vi "Initialize Configuration.vi"(8 "error in (no error)":errorcluster, 10 "framework configuration in":T1, 11 "VeriStand Data Sharing Framework in":refnum<class "VeriStand Data Sharing Framework.lvclass">) -> (0 "error out":errorcluster, 2 "framework configuration out":T1, 3 "VeriStand Data Sharing Framework out":refnum<class "VeriStand Data Sharing Framework.lvclass">)   [LabVIEW 2017, in "Data Sharing Custom Device Engine.lvlib" / "VeriStand Data Sharing Framework.lvclass"]
uses:
  VeriStand Data Sharing Framework.lvclass
  Builds/Data Sharing Framework/Current/Core/DSF Core.lvlibp/DSF Configuration API/Public/Controls/DSF Engine Framework Configuration.ctl
  Builds/Data Sharing Framework/Current/Core/DSF Core.lvlibp/DSF Configuration API/Public/Controls/DSF Engine Plugin Configuration.ctl
  Builds/Data Sharing Framework/Current/Core/DSF Core.lvlibp/DSF Configuration API/Public/Controls/DSF Timing Info.ctl
  Builds/Data Sharing Framework/Current/Core/DSF Core.lvlibp/DSF Configuration API/Public/Controls/DSF Engine Plugin Thread Configuration.ctl
  Builds/Data Sharing Framework/Current/Core/DSF Core.lvlibp/DSF Configuration API/Public/Controls/DSF Settings Info.ctl
  Builds/Data Sharing Framework/Current/Core/DSF Core.lvlibp/DSF Configuration API/Public/Controls/DSF Engine Transfer Group Configuration.ctl
  Builds/Data Sharing Framework/Current/Core/DSF Core.lvlibp/DSF Configuration API/Public/Controls/DSF Direction.ctl
  Builds/Data Sharing Framework/Current/Core/DSF Core.lvlibp/DSF Configuration API/Public/Controls/DSF Engine Transfer Configuration.ctl
  Builds/Data Sharing Framework/Current/Core/DSF Core.lvlibp/DSF Configuration API/Public/Controls/DSF Byte Order.ctl
  Builds/Data Sharing Framework/Current/Core/DSF Core.lvlibp/DSF Configuration API/Public/Controls/DSF Engine Channel Configuration.ctl
  Builds/Data Sharing Framework/Current/Core/DSF Core.lvlibp/DSF Configuration API/Public/Controls/DSF Data Type.ctl
  VeriStand Data Sharing Framework.lvclass/VeriStand Data Sharing Framework.ctl
  <vilib>/NI Veristand/Custom Device API/Data Access Type.ctl
  Builds/Data Sharing Framework/Current/Core/DSF Core.lvlibp/DSF Configuration API/Public/Channel Count (Transfer).vi
  <vilib>/NI Veristand/Custom Device API/Custom Device API.lvlib
  Builds/Data Sharing Framework/Current/Core/DSF Core.lvlibp
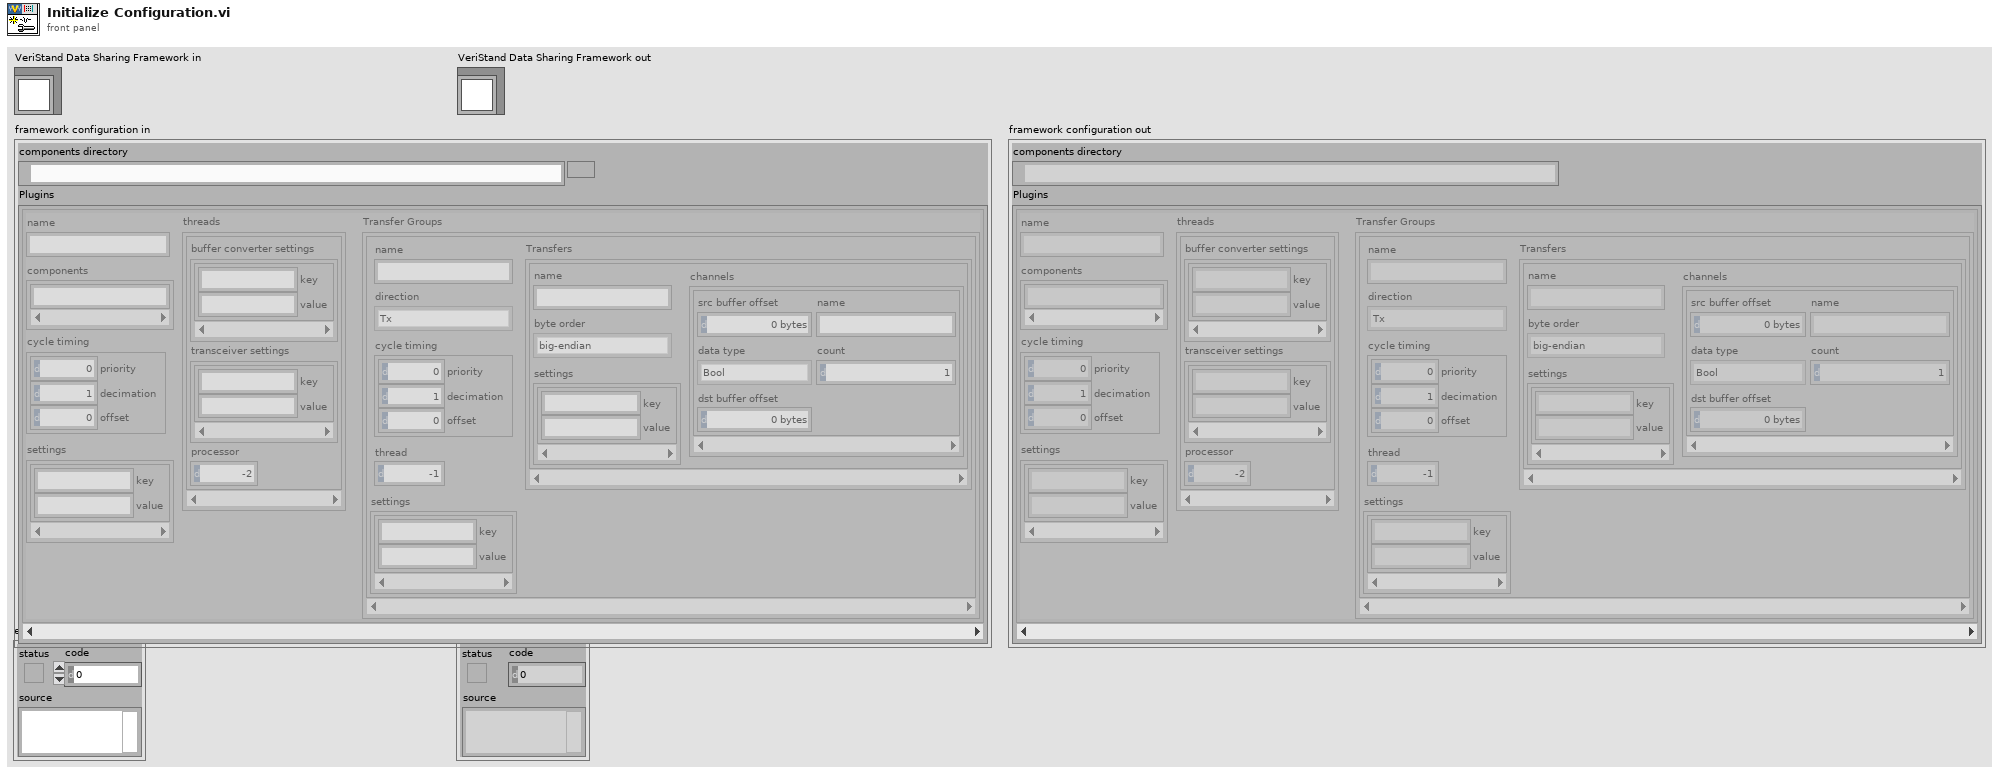
[diagram p1: front panel]
types:
  T1 = typedef "DSF Core.lvlibp/DSF Engine Framework Configuration.ctl" = cluster{"components directory":path, "Plugins":T2[]}
  T2 = typedef "DSF Core.lvlibp/DSF Engine Plugin Configuration.ctl" = cluster{"name":string, "components":string[], "cycle timing":T3, "threads":T4[], "Transfer Groups":T6[], "settings":T5}
  T3 = typedef "DSF Core.lvlibp/DSF Timing Info.ctl" = cluster{"priority":u64, "decimation":u64, "offset":u64}
  T4 = typedef "DSF Core.lvlibp/DSF Engine Plugin Thread Configuration.ctl" = cluster{"buffer converter settings":T5, "transceiver settings":T5, "processor":i32}
  T5 = typedef "DSF Core.lvlibp/DSF Settings Info.ctl" = cluster{"key":string, "value":string}[]
  T6 = typedef "DSF Core.lvlibp/DSF Engine Transfer Group Configuration.ctl" = cluster{"name":string, "direction":T7, "cycle timing":T3, "thread":i32, "settings":T5, "Transfers":T8[]}
  T7 = typedef "DSF Core.lvlibp/DSF Direction.ctl" = enum8{"Tx", "Rx"}
  T8 = typedef "DSF Core.lvlibp/DSF Engine Transfer Configuration.ctl" = cluster{"name":string, "byte order":T9, "channels":T10[], "settings":T5}
  T9 = typedef "DSF Core.lvlibp/DSF Byte Order.ctl" = enum8{"big-endian", "little-endian"}
  T10 = typedef "DSF Core.lvlibp/DSF Engine Channel Configuration.ctl" = cluster{"src buffer offset":u64, "name":string, "data type":T11, "count":u64, "dst buffer offset":u64}
  T11 = typedef "DSF Core.lvlibp/DSF Data Type.ctl" = enum8{"Bool", "SGL", "DBL", "I8", "I16", "I32", "I64", "U8", "U16", "U32", "U64"}
  T12 = typedef "Custom Device API.lvlib/Data Access Type.ctl" = enum16{"Read", "Write"}
  T13 = typedef "Custom Device API.lvlib/Custom Device Item Ref.ctl" = u64
  T14 = typedef "Custom Device API.lvlib/Block Data Reference.ctl" = cluster{"Data Reference":T15, "Offset":u64, "Length":u64}
  T15 = typedef "Custom Device API.lvlib/Data Reference.ctl" = i32
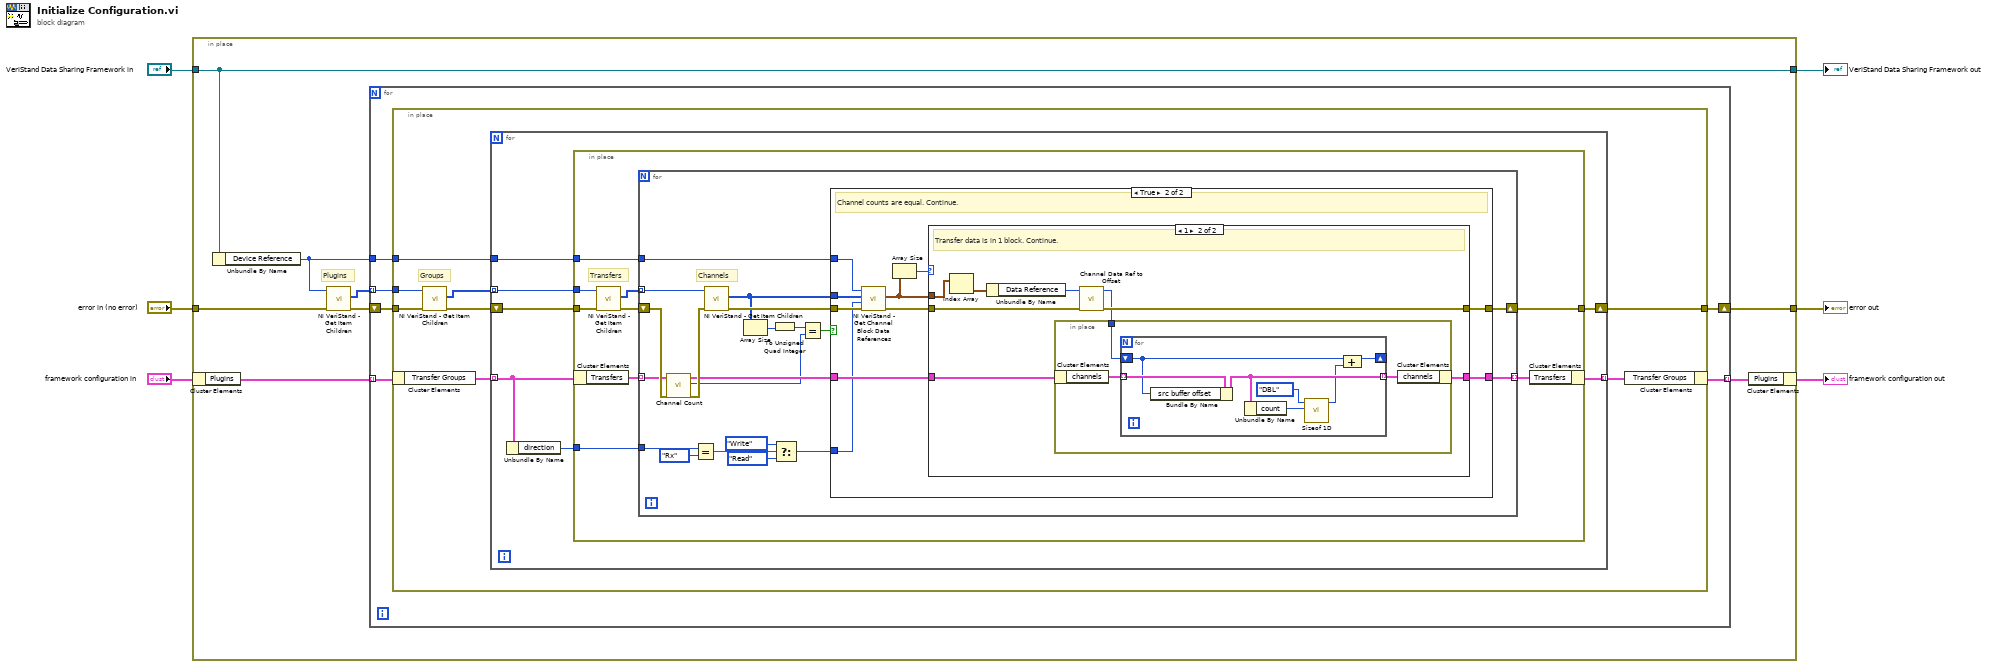
[diagram p0: block diagram]
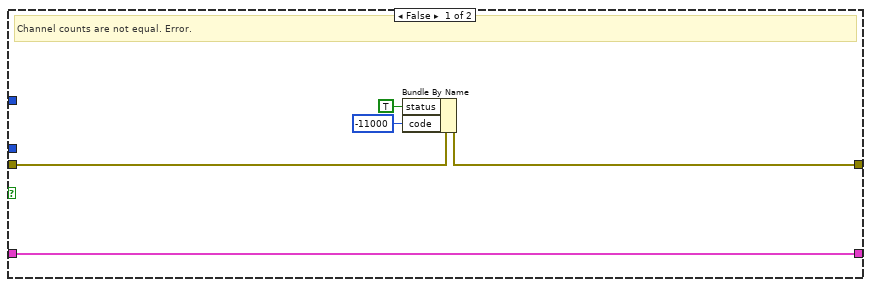
[diagram p2: hidden frame]
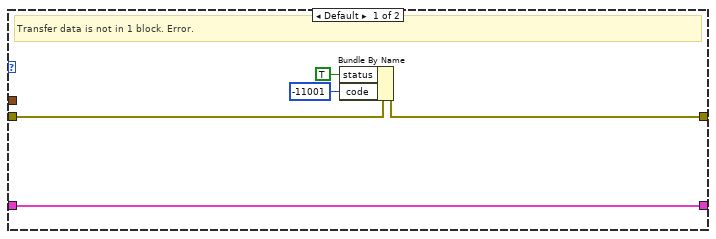
[diagram p3: hidden frame]
diagram:
  n1 = in-place {
    in-place-border: "VeriStand Data Sharing Framework in" -> [w13]
    in-place-border: [w13] -> w5
    in-place-border: "error in (no error)" -> [w8]
    in-place-border: [w7] -> w1
    # "Plugins"
    n2 = in-place-cluster #1("framework configuration in") -> ("Plugins"=w12:T2[])
    n3 = Unbundle By Name(w13) -> ("Device Reference"=w10:T13)
    n4 = call <vilib>:"NI VeriStand - Get Item Children.vi"("error in (no error)"=w8, "Item Ref in"=w10) -> ("error out"=w9:errorcluster, "Child Refs"=w14:T13[])  [unwired: 6 in, 2 out]
    n5 = for {
      tunnel: w14 -> [w18] mode=indexing
      tunnel: w12 -> [w20] mode=indexing
      tunnel: [w19] -> w11 mode=indexing
      tunnel: w10 -> [w17]
      shift-right: [w15] -> w7
      shift-left: w9 -> [w16]
      n6 = in-place {
        in-place-border: w18 -> [w26]
        in-place-border: w17 -> [w24]
        in-place-border: w16 -> [w23]
        in-place-border: [w21] -> w15
        # "Groups"
        n7 = in-place-cluster #2(w20) -> ("Transfer Groups"=w28:T6[])
        n8 = call <vilib>:"NI VeriStand - Get Item Children.vi"("error in (no error)"=w23, "Item Ref in"=w26) -> ("error out"=w22:errorcluster, "Child Refs"=w25:T13[])  [unwired: 6 in, 2 out]
        n9 = for {
          tunnel: w28 -> [w33] mode=indexing
          tunnel: [w35] -> w27 mode=indexing
          tunnel: w25 -> [w34] mode=indexing
          tunnel: w24 -> [w31]
          shift-right: [w29] -> w21
          shift-left: w22 -> [w30]
          n10 = Unbundle By Name(w33) -> ("direction"=w32:T7)
          n11 = in-place {
            in-place-border: w34 -> [w44]
            in-place-border: w32 -> [w41]
            in-place-border: w31 -> [w40]
            in-place-border: w30 -> [w39]
            in-place-border: [w37] -> w29
            # "Transfers"
            n12 = in-place-cluster #3(w33) -> ("Transfers"=w43:T8[])
            n13 = call <vilib>:"NI VeriStand - Get Item Children.vi"("error in (no error)"=w39, "Item Ref in"=w44) -> ("error out"=w38:errorcluster, "Child Refs"=w42:T13[])  [unwired: 6 in, 2 out]
            n14 = for {
              tunnel: w43 -> [w47] mode=indexing
              tunnel: w42 -> [w64] mode=indexing
              tunnel: w41 -> [w62]
              tunnel: w40 -> [w55]
              shift-right: [w46] -> w37
              shift-left: w38 -> [w51]
              tunnel: [w45] -> w36 mode=indexing
              # "Channels"
              n15 = call-poly "Channel Count.vi"("error in (no error)"=w51, "Transfer Configuration in"=w47) -> ("error out"=w50:errorcluster, "total channel count"=w48:u64, "Transfer Configuration out"=w49:T8)  [unwired: 7 in]
              n16 = Equal?(x=w62, y=DSF_Direction."Rx") -> (x = y?=w60:bool)
              n17 = call <vilib>:"NI VeriStand - Get Item Children.vi"("error in (no error)"=w50, "Item Ref in"=w64) -> ("error out"=w53:errorcluster, "Child Refs"=w52:T13[])  [unwired: 6 in, 2 out]
              n18 = Array Size(array=w52) -> (size(s)=w63:i32)
              n19 = To Unsigned Quad Integer(1:w63) -> (0:w56:u64)
              n20 = Select(t=Data_Access_Type."Write" ("Access"), s=w60, f=Data_Access_Type."Read") -> (s? t:f=w54:T12)
              n21 = Equal?(x=w56, y=w48) -> (x = y?=w57:bool)
              n22 = case shown="True" w57 {
                tunnel: w52 -> [_ w79]
                tunnel: w55 -> [_ w78]
                tunnel: w54 -> [_ w73]
                tunnel: w49 -> [w69 w75]
                tunnel: w53 -> [w68 w74]
                tunnel: [w67 w71] -> w46
                tunnel: [w69 w70] -> w45
                frame False {
                  # "Channel counts are not equal. Error."
                  n23 = Bundle By Name(cluster=w68, "status"=TRUE, "code"=-11000) -> (w67:errorcluster)
                }
                frame True {
                  # "Channel counts are equal. Continue."
                  n24 = call <vilib>:"NI VeriStand - Get Channel Block Data References.vi"("error in (no error)"=w74, "Access"=w73, "Channel Refs"=w79, "Device Ref in"=w78) -> ("error out"=w72:errorcluster, "Block Data Refs"=w76:T14[])  [unwired: 4 in, 2 out]
                  n25 = Array Size(array=w76) -> (size(s)=w77:i32)
                  n26 = case shown="1" w77 {
                    tunnel: w76 -> [_ w92]
                    tunnel: w75 -> [w84 w87]
                    tunnel: w72 -> [w81 w89]
                    tunnel: [w80 w88] -> w71
                    tunnel: [w84 w85] -> w70
                    frame Default {
                      # "Transfer data is not in 1 block. Error."
                      n27 = Bundle By Name(cluster=w81, "status"=TRUE, "code"=-11001) -> (w80:errorcluster)
                    }
                    frame 1 {
                      # "Transfer data is in 1 block. Continue."
                      n28 = Index Array(array=w92) -> (element=w91:T14)  [unwired: 1 in]
                      n29 = Unbundle By Name(w91) -> ("Data Reference"=w90:T15)
                      n30 = call "Channel Data Ref to Offset.vi"("error in (no error)"=w89, "Channel Data Reference"=w90) -> ("error out"=w88:errorcluster, "channel offset"=w86:u64)  [unwired: 8 in]
                      n31 = in-place {
                        in-place-border: w86 -> [w93]
                        n32 = in-place-cluster #4(w87) -> ("channels"=w95:T10[])
                        n33 = for {
                          tunnel: w95 -> [w100] mode=indexing
                          tunnel: [w99] -> w94 mode=indexing
                          shift-right: [w97] -> _
                          shift-left: w93 -> [w96]
                          n34 = Bundle By Name(cluster=w100, "src buffer offset"=w96) -> (w99:T10)
                          n35 = Unbundle By Name(w99) -> ("count"=w102:u64)
                          n36 = call "Sizeof 1D.vi"("count"=w102, "data type"=DSF_Data_Type."DBL") -> ("size in bytes"=w98:u64)  [unwired: 9 in]
                          n37 = Compound Arithmetic op=ADD(w96, w98) -> (w97:u64)
                        }
                        n38 = in-place-cluster #4("channels"=w94) -> (w85:T8)
                      }
                    }
                  }
                }
              }
            }
            n39 = in-place-cluster #3("Transfers"=w36) -> (w35:T6)
          }
        }
        n40 = in-place-cluster #2("Transfer Groups"=w27) -> (w19:T2)
      }
    }
    n41 = in-place-cluster #1("Plugins"=w11) -> (→"framework configuration out":T1)
  }
  "error out" <- w1
  "VeriStand Data Sharing Framework out" <- w5
